vi "Save-Recall Set.vi"(5 "Memory Location (0)":i32(ring) items=["0", "1", "2", "3", "4", "5", "6", "7", "8", "9"], 7 "Operation (0: Save)":u16(ring) items=["Save", "Recall"], 8 "error in (no error)":errorcluster, 11 "VISA resource name":refnum<visa-resource-name>) -> (0 "error out":errorcluster, 3 "VISA resource name out":refnum<visa-resource-name>="COM")   [LabVIEW 2020, in "GPP.lvlib"]
uses:
  GPP.lvlib
  Function/VISA_COMMON.ctl
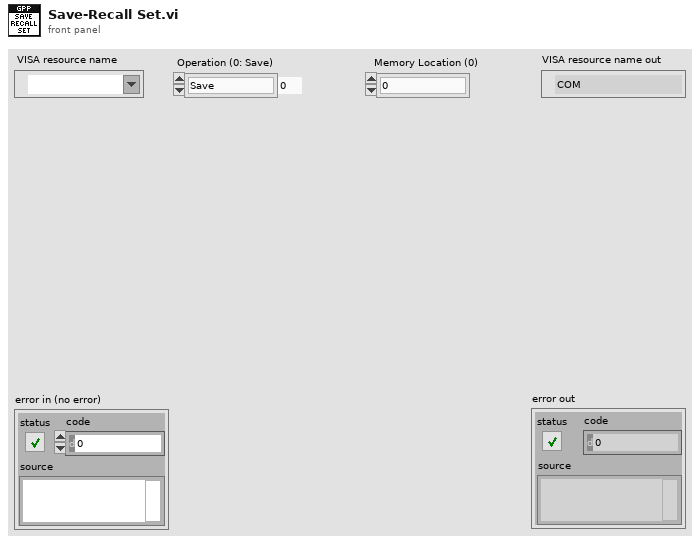
[diagram p1: front panel]
types:
  T1 = typedef "GPP.lvlib/VISA_COMMON.ctl" = enum16{"Initial", "Write CMD", "Read Result", "Read History", "Close"}
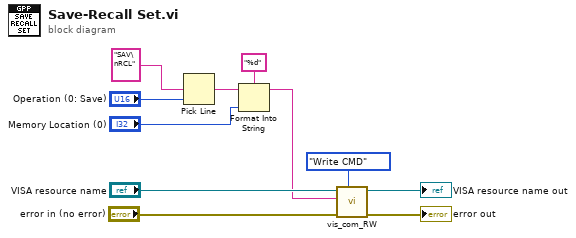
[diagram p0: block diagram]
diagram:
  n1 = Pick Line(multi-line string="SAV\nRCL", line index="Operation (0: Save)") -> (output string=w10:string)  [unwired: 1 out]
  n2 = Format Into String(format string="%d", initial string=w10, "Memory Location (0)") -> (resulting string=w3:string)  [unwired: 1 in, 1 out]
  n3 = call "vis_com_RW.vi"("Funciton"=VISA_COMMON."Write CMD", "error in (no error)"="error in (no error)", "CMD String"=w3, "VISA resource in"="VISA resource name") -> ("error out"=→"error out":errorcluster, "VISA resource out"=→"VISA resource name out":refnum<visa-resource-name>)  [unwired: 5 in, 1 out]
